vi "GD_GWID9F_info.vi"(7 "glue_id":string, 8 "error in (no error)":errorcluster, 10 "glue_3":sgl=2.5, 11 "DBlink":string="Driver={ODBC Driver 17 for SQL Server};Server=localhost\\SQLEXPRESS;Database=ZDX201;UID=labview;PWD=Dsa@54137926") -> (0 "error out":errorcluster)   [LabVIEW 2019]
uses:
  <vilib>/addons/database/Auxilliary.llb/DB Tools Format Datetime String (Time Stamp).vi
  <vilib>/addons/database/Connection.llb/DB Tools Open Connec (String).vi
  <vilib>/addons/database/NI_Database_API.lvlib
panel:
  out "Command 2":string="WHERE [id]=16"
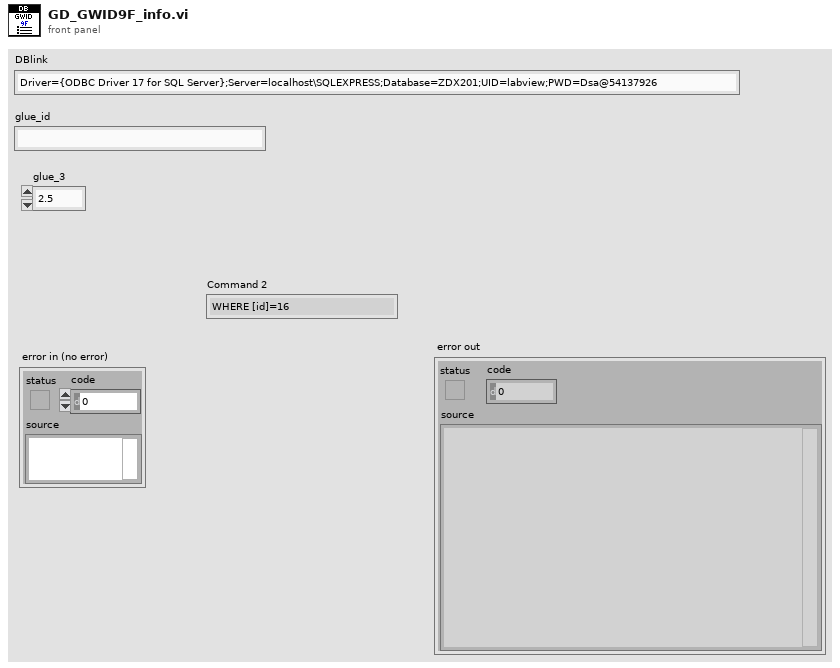
[diagram p1: front panel]
types:
  T1 = cluster{"glue_3":sgl, "update_time":timestamp, "time_finish_3":timestamp}
  T2 = typedef "NI_Database_API.lvlib/Conn ObjectReference.ctl" = refnum<k1>
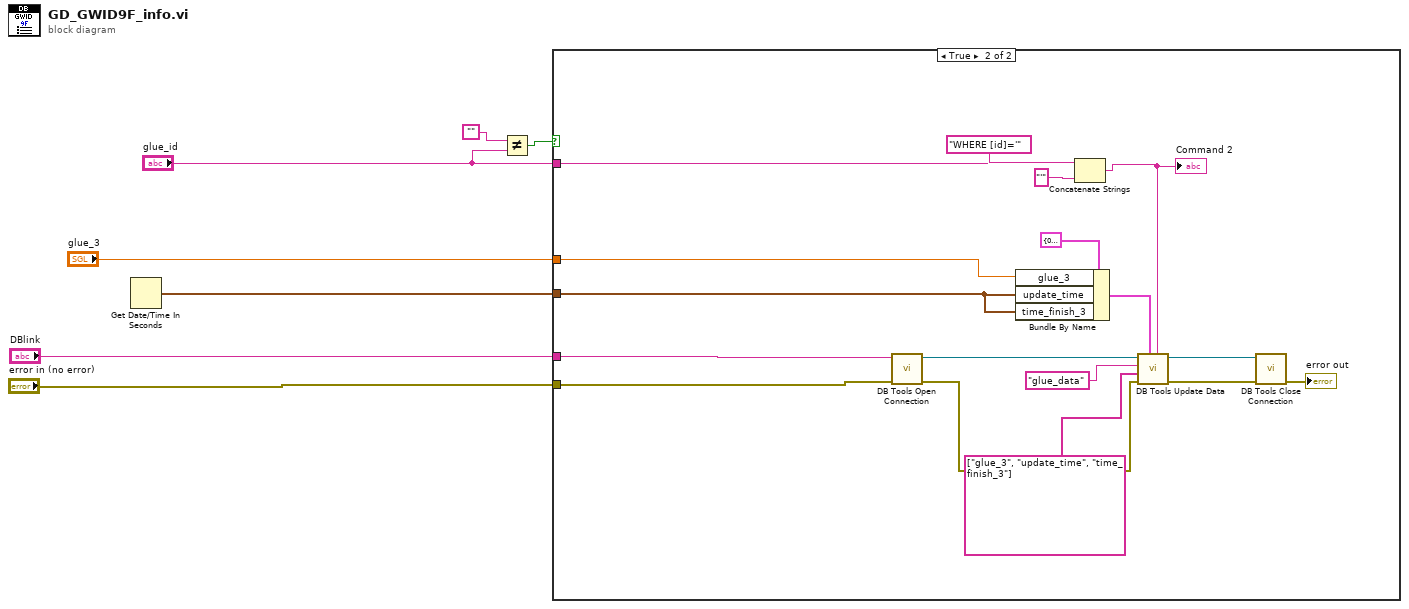
[diagram p0: block diagram]
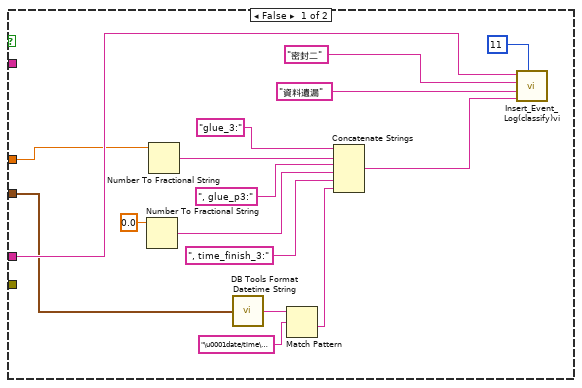
[diagram p2: hidden frame]
diagram:
  n1 = Get Date/Time In Seconds() -> (seconds since 1Jan1904=w7:timestamp)
  n2 = Not Equal?(x="", y="glue_id") -> (x != y?=w3:bool)
  n3 = case shown="True" w3 {
    tunnel: w7 -> [w9 w31]
    tunnel: "glue_3" -> [w10 w30]
    tunnel: "DBlink" -> [w11 w26]
    tunnel: "error in (no error)" -> [_ w25]
    tunnel: "glue_id" -> [_ w24]
    frame False {
      n4 = Number To Fractional String(number=0.0) -> (F-format string=w16:string)  [unwired: 3 in]
      n5 = Number To Fractional String(number=w10) -> (F-format string=w18:string)  [unwired: 3 in]
      n6 = call-poly <vilib>:"DB Tools Format Datetime String.vi"("time stamp"=w9) -> ("date/time string"=w20:string)
      n7 = Match Pattern(string=w20, regular expression="\u0001date/time\u0001" ("search string")) -> (after substring=w14:string)  [unwired: 1 in, 3 out]
      n8 = Concatenate Strings("glue_3:", w18, ", glue_p3:", w16, ", time_finish_3:", w14) -> (w13:string)
      n9 = call "Insert_Event_Log(classify)vi.vi"("classify"=i16 11, "data"=w13, "message"="資料遺漏", "id"="密封二", "DBlink"=w11) -> ()  [unwired: 6 in, 1 out]
    }
    frame True {
      n10 = call-poly <vilib>:"DB Tools Open Connection.vi"("error in (no error)"=w25, "connection information"=w26) -> ("error out"=w39:errorcluster, "connection reference"=w32:T2)  [unwired: 6 in]
      n11 = Bundle By Name(cluster=T1 {"glue_3"=0.0, "update_time"=timestamp(0 s since 1904-01-01), "time_finish_3"=timestamp(0 s since 1904-01-01)}, "glue_3"=w30, "update_time"=w31, "time_finish_3"=w31) -> (w33:T1)
      n12 = Concatenate Strings("WHERE [id]='", w24, "'" ("string")) -> (w27:string)
      "Command 2" <- w27
      n13 = call <vilib>:"DB Tools Update Data.vi"("condition"=w27, "data"=w33, "error in (no error)"=w39, "columns"=string[] ["glue_3", "update_time", "time_finish_3"], "table"="glue_data", "connection reference"=w32) -> ("error out"=w40:errorcluster, "connection reference out"=w38:T2)  [unwired: 4 in]
      n14 = call <vilib>:"DB Tools Close Connection.vi"("error in (no error)"=w40, "connection reference"=w38) -> ("error out"=→"error out":errorcluster)  [unwired: 5 in]
    }
  }
